vi "Report Error.vi"(5 "Callchain (T)":bool=TRUE, 7 "Context (None)":string, 8 "error in (no error)":errorcluster, 11 "EventLoggingService in":refnum<class "EventLoggingService.lvclass">) -> (0 "error out":errorcluster, 3 "EventLoggingService out":refnum<class "EventLoggingService.lvclass">)   [LabVIEW 2020, in "Vecto.lvlib" / "EventLoggingService.lvclass"]
uses:
  EventLoggingService.lvclass
  EventLoggingService.lvclass/EventLoggingService.ctl
  EventLogHandler/EventLogHandler.lvclass
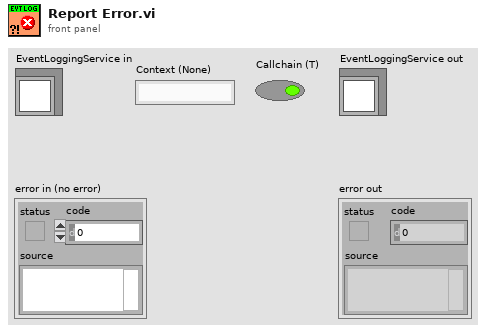
[diagram p1: front panel]
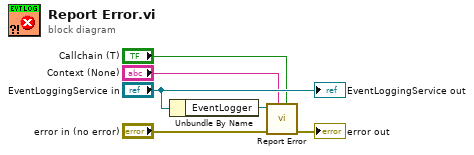
[diagram p0: block diagram]
diagram:
  n1 = Unbundle By Name("EventLoggingService in") -> ("EventLogger"=w5:refnum<class "EventLogHandler.lvclass">)
  n2 = call "Report Error.vi"("Callchain (T)"="Callchain (T)", "Context (None)"="Context (None)", "error in (no error)"="error in (no error)", "EventLogHandler in"=w5) -> ("error out"=→"error out":errorcluster)  [unwired: 7 in]
  "EventLoggingService out" <- "EventLoggingService in"
